vi "Pre Launch Init.vi"(11 "GarphView in":refnum<class "GarphView.lvclass">) -> (0 "error out":errorcluster, 3 "GarphView out":refnum<class "GarphView.lvclass">)   [LabVIEW 2020, in "GarphView.lvlib" / "GarphView.lvclass"]
uses:
  GarphView.lvclass
  GarphView.lvclass/GarphView.ctl
  <vilib>/gpm_packages/@cs/mva-viewable/Source/IViewable/IViewable/IViewable.lvclass
  <vilib>/gpm_packages/@cs/lookup-table/Source/LookupTable/LookupTable.lvclass
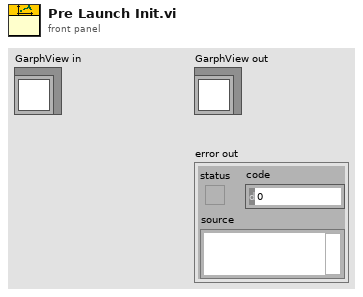
[diagram p1: front panel]
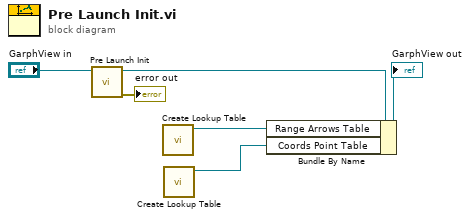
[diagram p0: block diagram]
diagram:
  n1 = call-parent "Pre Launch Init.vi"("IViewable in"="GarphView in") -> ("error out"=→"error out":errorcluster, "IViewable out"=w5:refnum<class "GarphView.lvclass">)  [unwired: 9 in]
  n2 = call <vilib>:"Create Lookup Table.vi"() -> ("LookupTable Reference"=w2:refnum<data-value>)  [unwired: 10 in, 1 out]
  n3 = call <vilib>:"Create Lookup Table.vi"() -> ("LookupTable Reference"=w1:refnum<data-value>)  [unwired: 10 in, 1 out]
  n4 = Bundle By Name(cluster=w5, "Range Arrows Table"=w2, "Coords Point Table"=w1) -> (→"GarphView out":refnum<class "GarphView.lvclass">)
